vi "Close.vi"(8 "error in (no error)":errorcluster, 11 "TDS 2000 in":refnum<class "TDS 2000.lvclass">) -> (0 "error out":errorcluster, 3 "TDS 2000 out":refnum<class "TDS 2000.lvclass">)   [LabVIEW 2020, in "Oscilloscope.lvlib" / "TDS 2000.lvclass"]
uses:
  TDS 2000.lvclass
  C:/Users/ronad/Osciloscopio/Osciloscopio DQMH/Libraries/Oscilloscope/Clases/Osciloscopio/Osciloscopio.lvclass
  Osciloscopio/Osciloscopio.lvclass/Osciloscopio.ctl
  Osciloscopio/Read COM.vi
  <instrlib>/Tektronix TDS 200 1000 2000 Series/Tektronix TDS 200 1000 2000 Series.lvlib
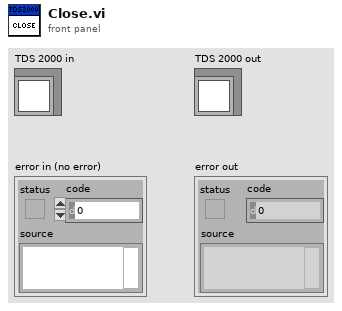
[diagram p1: front panel]
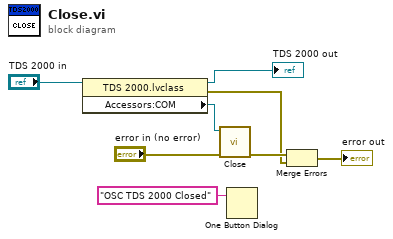
[diagram p0: block diagram]
diagram:
  n1 = property class="TDS 2000.lvclass"(reference="TDS 2000 in") -> (reference out=→"TDS 2000 out":refnum<class "TDS 2000.lvclass">, error out=w2:errorcluster, "Accessors:COM"=w8:refnum<visa-resource-name>)  [unwired: 1 in]
  n2 = call <instrlib>:"Close.vi"("error in (no error)"="error in (no error)", "VISA resource name"=w8) -> ("error out"=w7:errorcluster)  [unwired: 9 in]
  n3 = One Button Dialog(message="OSC TDS 2000 Closed") -> ()  [unwired: 1 in, 1 out]
  n4 = Merge Errors(w7, w2) -> (→"error out":errorcluster)
